vi "Add Plugin Sections.vi"(8 "error in (no error)":errorcluster, 10 "Framework Configuration":refnum<class "Framework Configuration.lvclass">=refnum, 11 "Item Ref in":T1 format="%.0x") -> (0 "error out":errorcluster, 3 "Item Ref out":T1 format="%.0x")   [LabVIEW 2021, in "DSF System Explorer.lvlib"]
uses:
  DSF System Explorer.lvlib
  Shared/DSF Shared.lvlib
  Shared/Thread Page GUID.vi
  Shared/Plugin Page GUID.vi
  Shared/Group Page GUID.vi
  Shared/Transfer Page GUID.vi
  <vilib>/NI VeriStand/Custom Device API/Custom Device Item Ref.ctl
  <vilib>/NI VeriStand/Custom Device API/Custom Device API.lvlib
  Includes/DSF Core.lvlibp/Classes/Configuration/Core/Framework/Framework Configuration.lvclass
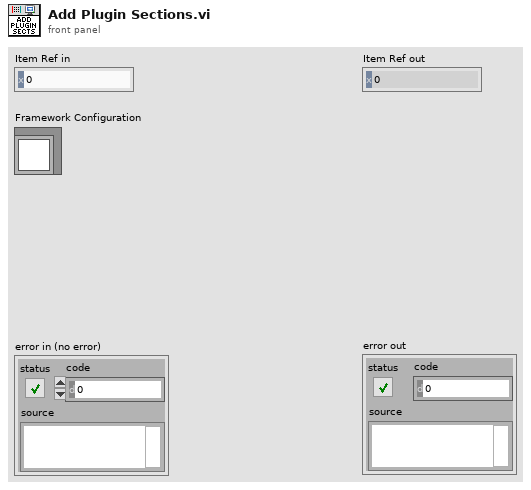
[diagram p1: front panel]
types:
  T1 = typedef "Custom Device API.lvlib/Custom Device Item Ref.ctl" = u64
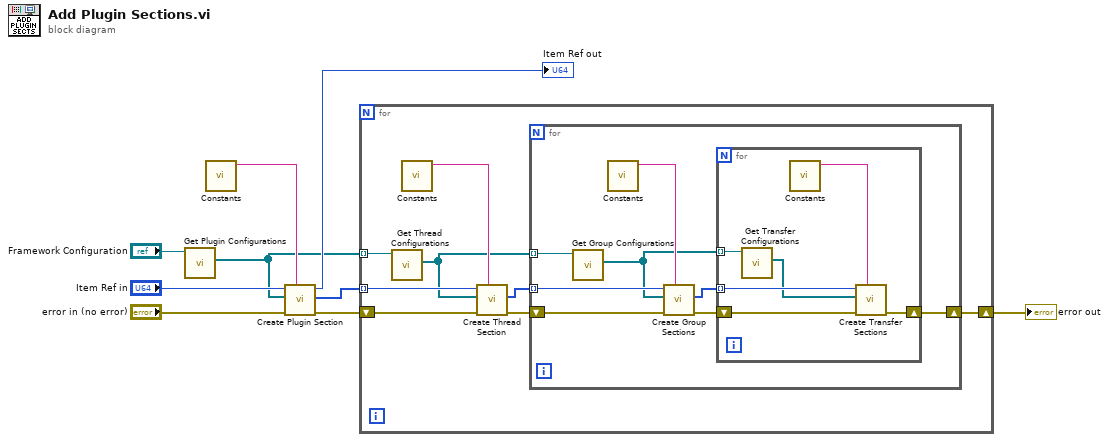
[diagram p0: block diagram]
diagram:
  n1 = call "Get Plugin Configurations.vi"("Framework Configuration in"="Framework Configuration") -> ("Plugin Configurations"=w1:refnum<class "Plugin Configuration.lvclass">[])  [unwired: 8 in, 2 out]
  n2 = call-poly "Constants.vi"() -> ("Plugin GUID"=w4:string)  [unwired: 11 in]
  n3 = call "Create Plugin Section.vi"("GUID (Default Section)"=w4, "error in (no error)"="error in (no error)", "Plugin Configurations"=w1, "Item Ref in"="Item Ref in") -> ("error out"=w8:errorcluster, "Plugin Section refs"=w6:T1[], "Item Ref out"=→"Item Ref out":T1)  [unwired: 5 in]
  n4 = for {
    tunnel: w6 -> [w15] mode=indexing
    tunnel: w1 -> [w11] mode=indexing
    shift-right: [w17] -> w7
    shift-left: w8 -> [w16]
    n5 = call "Get Thread Configurations.vi"("Plugin Configuration in"=w11) -> ("Thread Configurations"=w10:refnum<class "Thread Configuration.lvclass">[])  [unwired: 8 in, 2 out]
    n6 = call-poly "Constants.vi"() -> ("Thread GUID"=w12:string)  [unwired: 11 in]
    n7 = call "Create Thread Section.vi"("GUID (Default Section)"=w12, "error in (no error)"=w16, "Thread Configurations"=w10, "Item Ref in"=w15) -> ("error out"=w13:errorcluster, "Thread Section refs"=w14:T1[])  [unwired: 5 in, 1 out]
    n8 = for {
      shift-right: [w23] -> w17
      shift-left: w13 -> [w21]
      tunnel: w14 -> [w25] mode=indexing
      tunnel: w10 -> [w19] mode=indexing
      n9 = call "Get Group Configurations.vi"("Thread Configuration in"=w19) -> ("Group Configurations"=w18:refnum<class "Group Configuration.lvclass">[])  [unwired: 8 in, 2 out]
      n10 = call-poly "Constants.vi"() -> ("Group GUID"=w20:string)  [unwired: 11 in]
      n11 = call "Create Group Sections.vi"("GUID (Default Section)"=w20, "error in (no error)"=w21, "Group Configurations"=w18, "Item Ref in"=w25) -> ("error out"=w24:errorcluster, "Group Section refs"=w22:T1[])  [unwired: 5 in, 1 out]
      n12 = for {
        shift-right: [w30] -> w23
        shift-left: w24 -> [w31]
        tunnel: w22 -> [w28] mode=indexing
        tunnel: w18 -> [w27] mode=indexing
        n13 = call "Get Transfer Configurations.vi"("Group Configuration in"=w27) -> ("Transfer Configurations"=w26:refnum<class "Transfer Configuration.lvclass">[])  [unwired: 8 in, 2 out]
        n14 = call-poly "Constants.vi"() -> ("Transfer GUID"=w29:string)  [unwired: 11 in]
        n15 = call "Create Transfer Sections.vi"("GUID (Default Section)"=w29, "error in (no error)"=w31, "Transfer Configurations"=w26, "Item Ref in"=w28) -> ("error out"=w30:errorcluster)  [unwired: 5 in, 2 out]
      }
    }
  }
  "error out" <- w7
